vi "Wait Client Loops Running Values.vi"(8 "error in (no error)":errorcluster, 9 "Value":bool, 11 "TCPMessaging in":refnum<class "TCPMessaging.lvclass">) -> (0 "error out":errorcluster, 3 "TCPMessaging out":refnum<class "TCPMessaging.lvclass">)   [LabVIEW 2020, in "Vecto.lvlib" / "TCPMessaging.lvclass"]
uses:
  TCPMessaging.lvclass
  TCPMessaging.lvclass/TCPMessaging.ctl
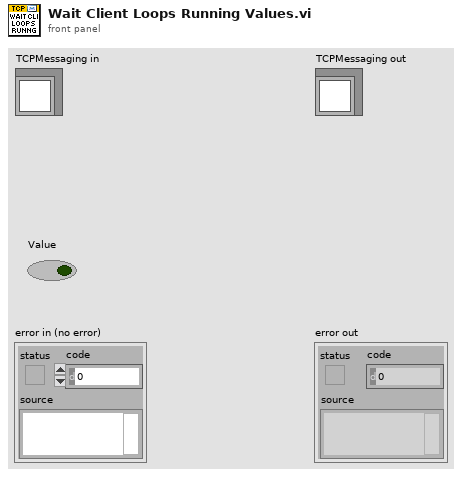
[diagram p1: front panel]
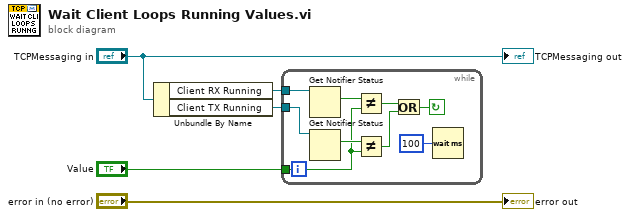
[diagram p0: block diagram]
diagram:
  n1 = Unbundle By Name("TCPMessaging in") -> ("Client RX Running"=w4:refnum<notifier>, "Client TX Running"=w3:refnum<notifier>)
  n2 = while {
    tunnel: w4 -> [w13]
    tunnel: w3 -> [w14]
    tunnel: "Value" -> [w8]
    stop <- w12 continue-if-true
    n3 = Get Notifier Status(notifier=w13) -> (current notification=w10:bool)  [unwired: 1 in, 4 out]
    n4 = Get Notifier Status(notifier=w14) -> (current notification=w9:bool)  [unwired: 1 in, 4 out]
    n5 = Not Equal?(x=w10, y=w8) -> (x != y?=w6:bool)
    n6 = Not Equal?(x=w9, y=w8) -> (x != y?=w7:bool)
    n7 = Or(x=w6, y=w7) -> (x .or. y?=w12:bool)
    n8 = Wait (ms)(milliseconds to wait=u32 100) -> ()  [unwired: 1 out]
  }
  "error out" <- "error in (no error)"
  "TCPMessaging out" <- "TCPMessaging in"
